vi "gen channels from bitfile action.vi"(8 "error in":errorcluster, 9 "user event":T1, 10 "engine configuration in":refnum<class "engine configuration.lvclass">, 11 "io configuration in":refnum<class "io configuration.lvclass">) -> (0 "error out":errorcluster, 2 "engine configuration out":refnum<class "engine configuration.lvclass">, 3 "io configuration out":refnum<class "io configuration.lvclass">)   [LabVIEW 2015, in "io editor node.lvclass"]
uses:
  io editor node.lvclass
  <vilib>/NI/Module Execution Interface/Engine Configuration/engine configuration.lvclass
  <vilib>/NI/Configuration Framework/Node/UserEventRef.ctl
  <vilib>/NI/Configuration Framework/Controls/EventCluster.ctl
  configuration/io configuration.lvclass
  configuration/io configuration.lvclass/io configuration.ctl
  <vilib>/NI/Configuration Framework/serializable configuration/NISE_CEF_serializable configuration.lvclass/NISE_CEF_serializable configuration.ctl
  table line.ctl
  <vilib>/NI/Tag Bus Module Framework/channel/TBM channel.lvclass
  <vilib>/Utility/LVClass/Get LV Class Name.vi
  <vilib>/NI/Configuration Framework/error generator/NISE_error generator.vi
  <vilib>/NI/Configuration Framework/NISE_CEF_TreeControl.lvlib
  <vilib>/NI/Configuration Framework/serializable configuration/NISE_CEF_serializable configuration.lvclass
  <vilib>/NI/Configuration Framework/Node/NISE_CEF_Node.lvclass
panel:
  out "strings":string[][](array[string])
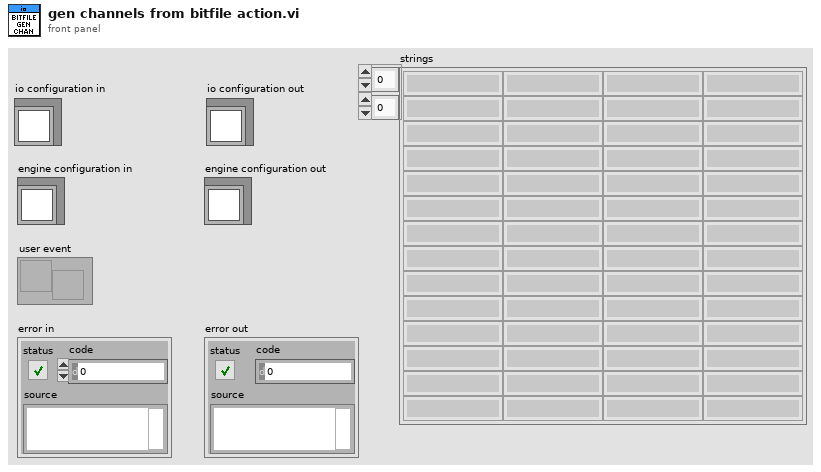
[diagram p1: front panel]
types:
  T1 = typedef "NISE_CEF_Node.lvclass/UserEventRef.ctl" = refnum<user-event>
  T2 = typedef "NISE_CEF_TreeControl.lvlib/EventCluster.ctl" = cluster{"command":string, "data":string}
  T3 = typedef "io editor node.lvclass/table line.ctl" = cluster{"channel":refnum<class "TBM channel.lvclass">, "tag name":string}
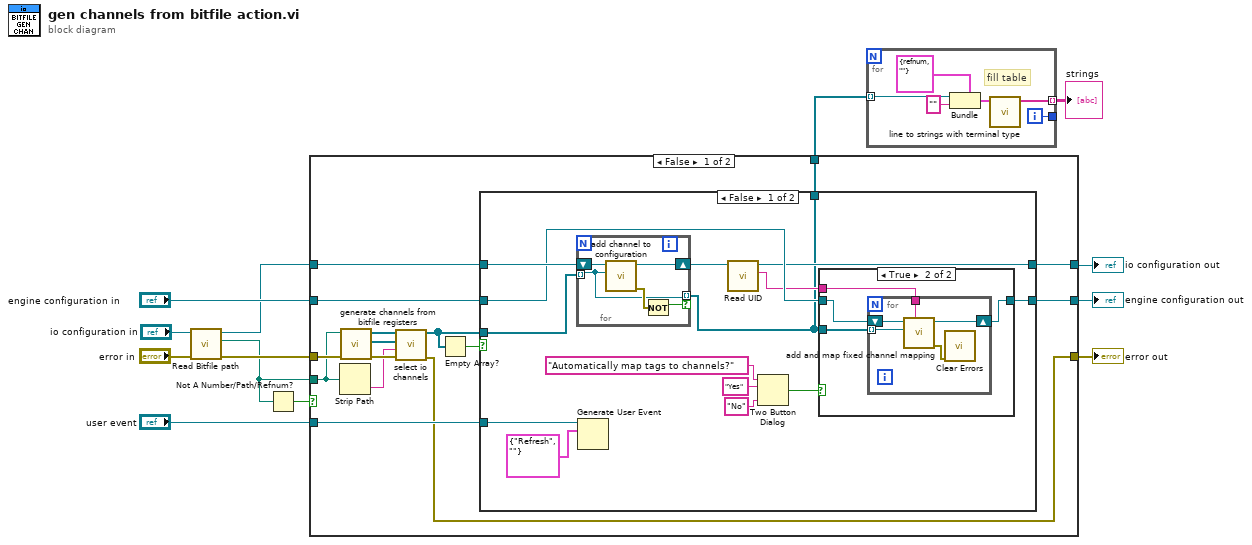
[diagram p0: block diagram]
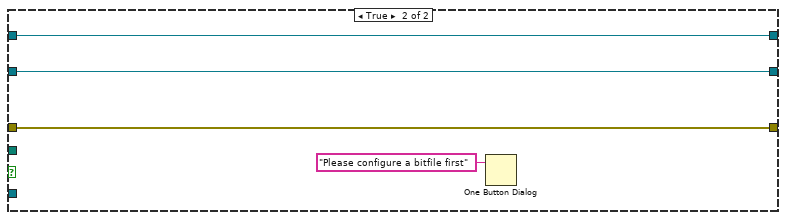
[diagram p4: hidden frame]
diagram:
  n1 = call "Read Bitfile path.vi"("error in (no error)"="error in", "io configuration in"="io configuration in") -> ("error out"=w5:errorcluster, "Bitfile path"=w3:path, "io configuration out"=w7:refnum<class "io configuration.lvclass">)  [unwired: 7 in]
  n2 = Not A Number/Path/Refnum?(number/path/refnum=w3) -> (NaN/Path/Refnum?=w10:bool)
  n3 = case shown="False" w10 {
    tunnel: w5 -> [w21 w61]
    tunnel: w7 -> [w28 w62]
    tunnel: [w26 w63] -> w13
    tunnel: "engine configuration in" -> [w27 w63]
    tunnel: [w24 w62] -> w9
    tunnel: [w22 w61] -> w4
    tunnel: w3 -> [w18 _]
    tunnel: "user event" -> [w25 _]
    tunnel: [w14 _] -> w1
    frame False {
      n4 = Strip Path(path=w18) -> (name=w17:string)  [unwired: 1 out]
      n5 = call "generate channels from bitfile registers.vi"("error in"=w21, "bitfilefile path"=w18) -> ("error out"=w20:errorcluster, "not supported channels"=w16:refnum<class "TBM channel.lvclass">[], "channels"=w19:refnum<class "TBM channel.lvclass">[])  [unwired: 7 in]
      n6 = call "select io channels.vi"("error in"=w20, "API Loaded"=w17, "not supported channels"=w16, "io channels"=w19) -> ("error out"=w22:errorcluster, "selected channels"=w15:refnum<class "TBM channel.lvclass">[])  [unwired: 6 in]
      n7 = Empty Array?(array=w15) -> (empty?=w23:bool)
      n8 = case shown="False" w23 {
        tunnel: w28 -> [w42 w59]
        tunnel: w15 -> [w41 _]
        tunnel: w27 -> [w36 w58]
        tunnel: [w35 w58] -> w26
        tunnel: w25 -> [w33 _]
        tunnel: [w31 w59] -> w24
        tunnel: [w29 _] -> w14
        frame False {
          n9 = for {
            tunnel: w41 -> [w54] mode=indexing
            shift-right: [w56] -> w37
            shift-left: w42 -> [w57]
            tunnel: [w54] -> w29 mode=indexing if=w53
            n10 = call "add channel to configuration.vi"("channel"=w54, "io configuration in"=w57) -> ("error out"=w55:errorcluster, "io configuration out"=w56:refnum<class "io configuration.lvclass">)  [unwired: 8 in]
            n11 = Not(x=w55) -> (.not. x?=w53:bool)
          }
          n12 = Generate User Event(user event=w33, event data cluster=T2 {"command"="Refresh", "data"=""} ("event data")) -> ()  [unwired: 2 in, 2 out]
          n13 = call <vilib>:"Read UID.vi"("configuration in"=w37) -> ("instance id"=w30:string, "configuration out"=w31:refnum<class "io configuration.lvclass">)  [unwired: 8 in, 1 out]
          n14 = Two Button Dialog(message="Automatically map tags to channels?", 1:"No" ("F button name (\"Cancel\")"), 2:"Yes" ("T button name (\"OK\")")) -> (T button?=w38:bool)
          n15 = case shown="True" w38 {
            tunnel: w36 -> [w43 w47]
            tunnel: [w43 w46] -> w35
            tunnel: w29 -> [_ w45]
            tunnel: w30 -> [_ w44]
            frame False {
            }
            frame True {
              n16 = for {
                shift-right: [w51] -> w46
                shift-left: w47 -> [w52]
                tunnel: w45 -> [w50] mode=indexing
                tunnel: w44 -> [w48]
                n17 = call <vilib>:"add and map fixed channel mapping.vi"("module instance"=w48, "fixed channel"=w50, "engine configuration in"=w52) -> ("error out"=w49:errorcluster, "engine configuration out"=w51:refnum<class "engine configuration.lvclass">)  [unwired: 7 in]
                n18 = call <vilib>:"Clear Errors.vi"("error in (no error)"=w49) -> ()  [unwired: 5 in, 2 out]
              }
            }
          }
        }
        frame True {
        }
      }
    }
    frame True {
      n19 = One Button Dialog(message="Please configure a bitfile first") -> ()  [unwired: 1 in, 1 out]
    }
  }
  "engine configuration out" <- w13
  "error out" <- w4
  "io configuration out" <- w9
  n20 = for {
    tunnel: w1 -> [w68] mode=indexing
    tunnel: [w65] -> w2 mode=indexing
    tunnel: [w64] -> _
    i -> [w64]
    # "fill table"
    n21 = Bundle(cluster=T3 {"channel"=refnum, "tag name"=""} ("line"), "channel"=w68, "tag name"="") -> (w66:T3)
    n22 = call "line to strings with terminal type.vi"("line"=w66) -> ("strings"=w65:string[])  [unwired: 10 in]
  }
  "strings" <- w2
